vi "Populate Method Results.vi"(8 "error in (no error)":errorcluster, 10 "Test Method Result":T1, 11 "Test Tree In":refnum<class "Test Result Tree V2.lvclass">) -> (0 "error out":errorcluster, 2 "Test Method Result Out":T1, 3 "Test Tree Out":refnum<class "Test Result Tree V2.lvclass">)   [LabVIEW 2020, in "Test Result Tree V2.lvclass"]
uses:
  Test Result Tree/Test Result Tree V2.lvclass
  C:/Git/astemes-lunit/source/Framework/Helper Classes/Test Tree/Test Tree.lvclass
  Framework/Result Types/Method Result/Method Result.ctl
  Result/Status.ctl
  Framework/Result Types/Assertion Result/Assertion Result.ctl
  Framework/Result Types/Assertion Result/Public/TypeDefs/Assertion Type.ctl
  Framework/Helper Classes/Test Tree/Test Tree.lvclass/Test Tree.ctl
  Test Result Tree/Test Result Tree V2.lvclass/Test Result Tree V2.ctl
  Framework/Helper Classes/Test Tree/Test Tree.lvclass
  Framework/Result Types/Method Result/Method Result.lvlib
  Framework/Result Types/Assertion Result/Assertion Result.lvlib
  Result/Result.lvlib
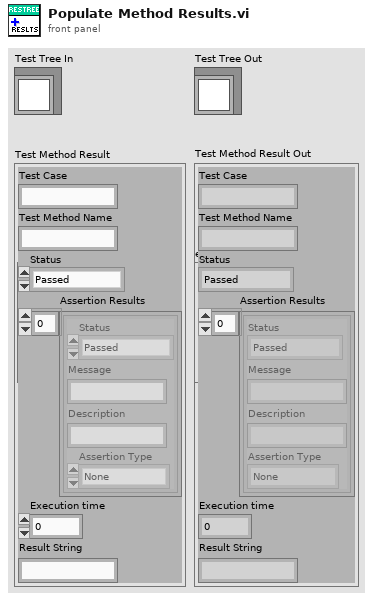
[diagram p1: front panel]
types:
  T1 = typedef "Method Result.lvlib/Method Result.ctl" = cluster{"Test Case":string, "Test Method Name":string, "Status":T2, "Assertion Results":T3[], "Execution time":dbl, "Result String":string}
  T2 = typedef "Result.lvlib/Status.ctl" = enum16{"Passed", "Failed", "Error", "Skipped", "Setup Error", "Broken", "Teardown Error"}
  T3 = typedef "Assertion Result.lvlib/Assertion Result.ctl" = cluster{"Status":T2, "Message":string, "Description":string, "Assertion Type":T4}
  T4 = typedef "Result.lvlib/Assertion Type.ctl" = enum16{"None", "Pass", "Fail", "Skip", "Pass if Equal", "Fail if Equal", "Pass if Error", "Fail if Error", "Pass if", "Fail if"}
  T5 = map{string, cluster{"Left Cell String":string, "Child Text":string[], "Item Indent":i32, "Child Only?":bool, "Glyph Index":i32}}
  T6 = typedef "Assertion Result.lvlib/Status.ctl" = enum16{"Pass", "Fail", "Error", "Skipped", "Setup Error", "Broken", "Teardown Error"}
  T7 = cluster{"Left Cell String":string, "Child Text":string[], "Item Indent":i32, "Child Only?":bool, "Glyph Index":i32}
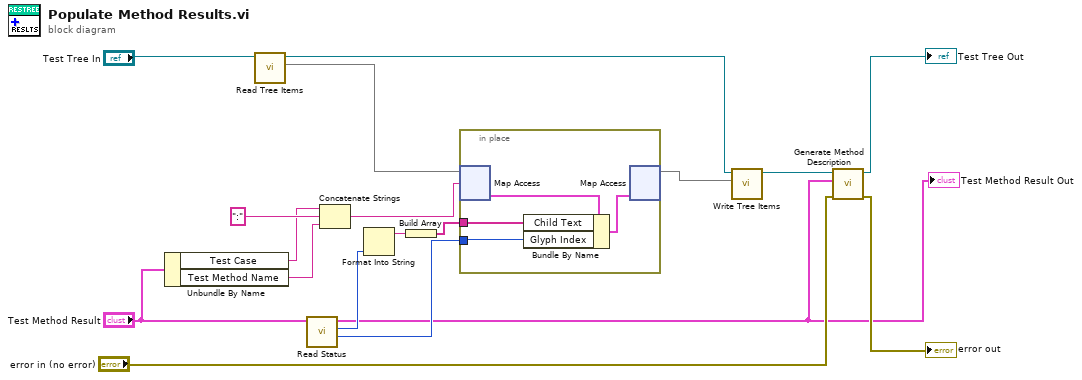
[diagram p0: block diagram]
diagram:
  n1 = Unbundle By Name("Test Method Result") -> ("Test Case"=w1:string, "Test Method Name"=w2:string)
  n2 = call "Read Tree Items.vi"("Test Tree In"="Test Tree In") -> ("Tree Items"=w8:T5, "Test Tree Out"=w10:refnum<class "Test Result Tree V2.lvclass">)  [unwired: 9 in]
  n3 = call "Read Status.vi"("Method Result In"="Test Method Result") -> ("Glyph Index"=w11:i32, "Status"=w17:T6, "Method Result Out"=w4:T1)  [unwired: 8 in]
  "Test Method Result Out" <- w4
  n4 = Concatenate Strings(w1, ":" ("string"), w2) -> (w13:string)
  n5 = Format Into String(w17) -> (resulting string=w16:string)  [unwired: 3 in, 1 out]
  n6 = Build Array(w16) -> (w12:string[])
  n7 = in-place {
    in-place-border: w12 -> [w22]
    in-place-border: w11 -> [w21]
    n8 = in-place-map #1(w8, w13) -> (w20:T7)  [unwired: 1 in, 1 out]
    n9 = Bundle By Name(cluster=w20, "Child Text"=w22, "Glyph Index"=w21) -> (w19:T7)
    n10 = in-place-map #1(w19) -> (w7:T5)  [unwired: 1 in, 2 out]
  }
  n11 = call "Write Tree Items.vi"("Tree Items"=w7, "Test Tree In"=w10) -> ("Test Tree Out"=w6:refnum<class "Test Result Tree V2.lvclass">)  [unwired: 9 in]
  n12 = call "Generate Method Description.vi"("error in (no error)"="error in (no error)", "Test Method Result In"=w4, "Test Tree In"=w6) -> ("error out"=→"error out":errorcluster, "Test Tree Out"=→"Test Tree Out":refnum<class "Test Result Tree V2.lvclass">)  [unwired: 7 in]
